vi "TB-Init Slack.vi"(0 "Allow Slack":bool, 2 "CtlRef":refnum<vi>) -> (4 "Slack":T1)   [LabVIEW 2020]
uses:
  Typedefs/TB-Slack State.ctl
  Typedefs/TB-User.ctl
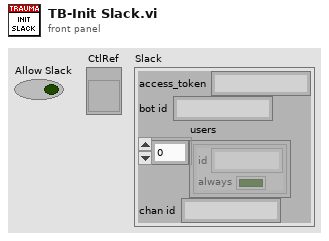
[diagram p1: front panel]
types:
  T1 = typedef "TB-Slack State.ctl" = cluster{"access_token":string, "bot id":string, "users":cluster{"id":string, "always":bool}[], "chan id":string}
  T2 = typedef "TB-User.ctl" = cluster{"name":string, "id":string, "notify on errors":bool}
  T3 = typedef "Slack-Configuration.ctl" = cluster{"app_id":string, "authed_user":cluster{"id":string}, "access_token":string, "bot_user_id":string, "team":cluster{"id":string, "name":string}, "bot channel":cluster{"id":string, "name":string}, "bot_user_name":string}
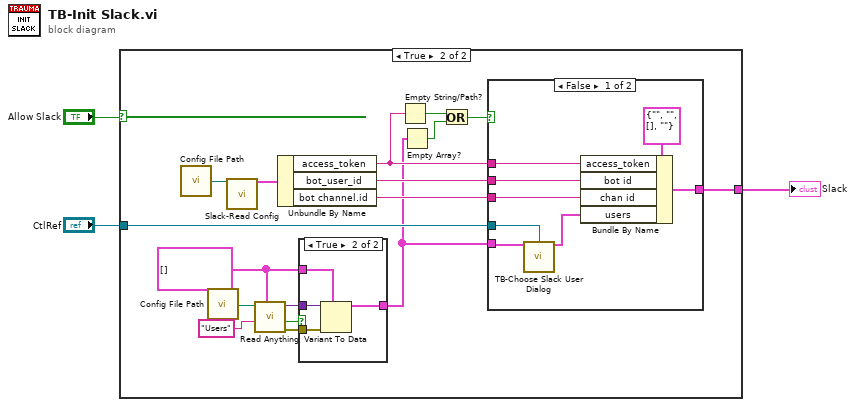
[diagram p0: block diagram]
diagram:
  n1 = case shown="True" "Allow Slack" {
    tunnel: [_ w18] -> w2
    tunnel: "CtlRef" -> [_ w15]
    frame False {
    }
    frame True {
      w6 = T2[] [] ("Array")
      n2 = call "Config File Path.vi"() -> ("Default config file name"=w20:path)  [unwired: 1 in]
      n3 = call "Config File Path.vi"() -> ("Default config file name"=w10:path)  [unwired: 1 in]
      n4 = call "Slack-Read Config.vi"("AppName"=w20) -> ("config"=w19:T3)  [unwired: 12 in, 2 out]
      n5 = call "Read Anything.vi"("Type of Anything"=w6, "Section Name (Name of \"Type of Anything\")"="Users" ("Section Name (Name of \"Anything\")"), "Path (dialog)"=w10) -> ("Error Out"=w7:errorcluster, "Found?"=w8:bool, "Anything"=w9:variant)  [unwired: 6 in]
      n6 = Unbundle By Name(w19) -> ("access_token"=w16:string, "bot_user_id"=w17:string, "bot channel.id"=w11:string)
      n7 = case shown="True" w8 {
        tunnel: w9 -> [_ w24]
        tunnel: w7 -> [_ w25]
        tunnel: w6 -> [w21 w23]
        tunnel: [w21 w22] -> w5
        frame False {
        }
        frame True {
          n8 = Variant To Data(error in=w25, type=w23, Variant=w24) -> (data=w22:T2[])  [unwired: 1 out]
        }
      }
      n9 = Empty String/Path?(string/path=w16) -> (empty?=w14:bool)
      n10 = Empty Array?(array=w5) -> (empty?=w13:bool)
      n11 = Or(x=w14, y=w13) -> (x .or. y?=w12:bool)
      n12 = case shown="False" w12 {
        tunnel: [w32 _] -> w18
        tunnel: w17 -> [w31 _]
        tunnel: w16 -> [w30 _]
        tunnel: w5 -> [w29 _]
        tunnel: w15 -> [w27 _]
        tunnel: w11 -> [w26 _]
        frame False {
          n13 = call "TB-Choose Slack User Dialog.vi"("users"=w29, "CtlRef"=w27) -> ("users"=w28:cluster{"id":string, "always":bool}[])  [unwired: 13 in]
          n14 = Bundle By Name(cluster=T1 {"access_token"="", "bot id"="", "users"=[], "chan id"=""} ("Slack"), "access_token"=w30, "bot id"=w31, "chan id"=w26, "users"=w28) -> (w32:T1)
        }
        frame True {
        }
      }
    }
  }
  "Slack" <- w2
